vi "Start.vi"(8 "error in (no error)":errorcluster, 11 "Vecto in":refnum<class "Vecto.lvclass">) -> (0 "error out":errorcluster, 3 "Vecto out":refnum<class "Vecto.lvclass">)   [LabVIEW 2020, in "Vecto.lvlib" / "Vecto.lvclass"]
uses:
  Vecto.lvclass
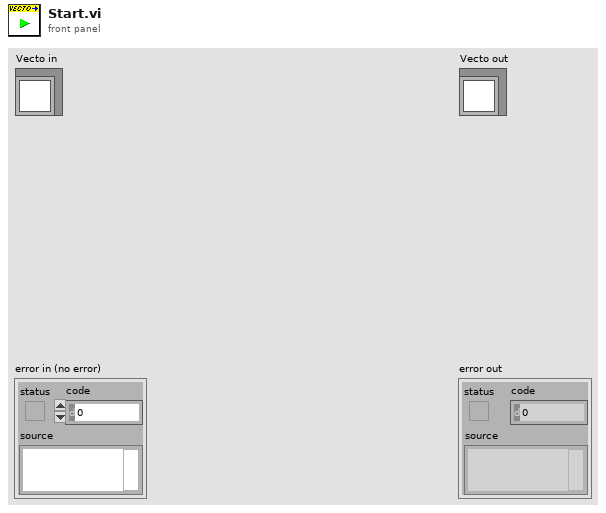
[diagram p1: front panel]
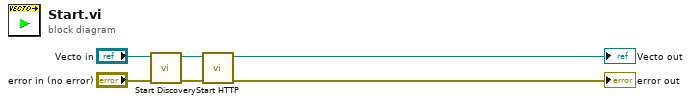
[diagram p0: block diagram]
diagram:
  n1 = call "Start Discovery.vi"("error in (no error)"="error in (no error)", "Vecto in"="Vecto in") -> ("error out"=w3:errorcluster, "Vecto out"=w1:refnum<class "Vecto.lvclass">)  [unwired: 8 in]
  n2 = call "Start HTTP.vi"("error in (no error)"=w3, "Vecto in"=w1) -> ("error out"=→"error out":errorcluster, "Vecto out"=→"Vecto out":refnum<class "Vecto.lvclass">)  [unwired: 8 in]
